vi "Load Subroutine Test Exec.vi"(4 "Path Builder":refnum<class "IPath Builder.lvclass">, 5 "Parallel in":refnum<class "Parallel.lvclass">, 6 "Persistence in":refnum<class "IPersist.lvclass">, 7 "Linked List ID":string, 8 "error in (no error)":errorcluster, 10 "Paths":path[](array[path]), 11 "Linked List Ref":refnum<data-value>) -> (0 "error out":errorcluster, 3 "Linked List Ref out":refnum<data-value>)   [LabVIEW 2017]
uses:
  Test Executive/ITestExecutive/ITest Executive.lvclass
  linked-list/Source/Linked List/Linked List Ref/Linked List Ref.lvclass
  b9c2613a-6aa9-4761-86d5-781f96568d67.vi
  Test Executive/TestExecutive Ref/TestExecutive Ref.lvclass
  cfb7364d-dae3-4f2b-ba87-61db7f054fd9.vi
  1f521296-bf4a-4187-b7fe-4ed0693accc0.vi
  8fd00299-f1f7-40b8-accc-d4ca8393805f.vi
  7c02b004-8b9d-45a5-be84-3e65cc974b1d.vi
  Test Executive Data Type/Test Executive.lvclass
  Custom Type Test Executive/Custom Type Test Executive.lvclass
  dc836278-d113-4003-92ad-fcb185286903.vi
  a563c450-6208-4c7f-b57f-94cea08b9ed5.vi
  6d463ee5-b5b8-463a-9b9c-645794412c76.vi
  data-type-serializer/source/Boolean/Boolean.lvclass
  data-type-serializer/source/String 1D/String 1D.lvclass
  Test Executive 1D Data Type/Test Executive 1D.lvclass
  C:/Users/jonmc/Documents/Git/Test Executive/gpm_packages/@cs/data-type-serializer/source/Data Type/Data Type.lvclass
  C:/Users/jonmc/Documents/Git/Test Executive/Source/Test Executive/ITestExecutive/ITest Executive.lvclass
  linked-list/Source/Linked List/ILinkedList/ILinked List.lvclass
  Path Builder/IPath Builder/IPath Builder.lvclass
  persistence/source/IPersist/IPersist.lvclass
  Parallel.lvclass
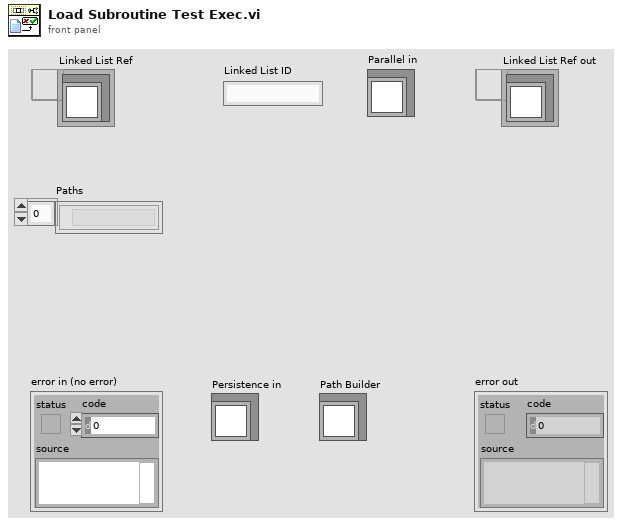
[diagram p1: front panel]
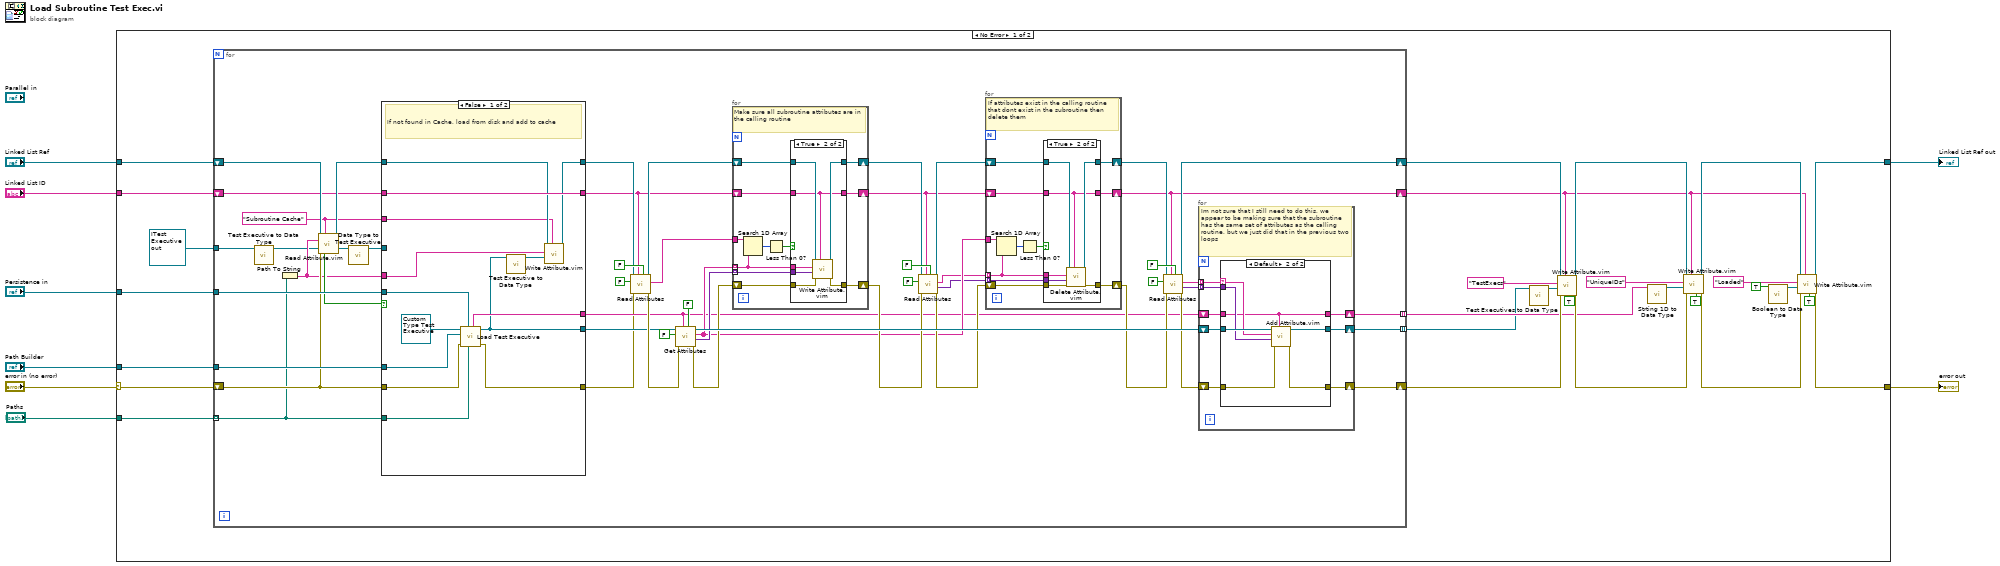
[diagram p0: block diagram]
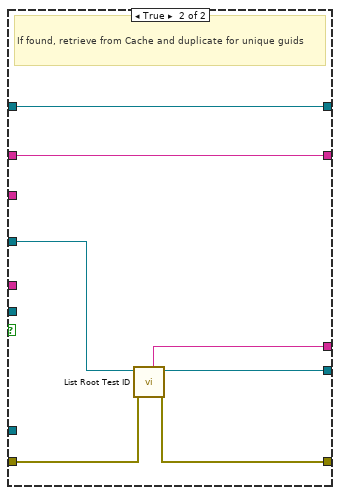
[diagram p2: hidden frame]
diagram:
  n1 = case shown="No Error" "error in (no error)" {
    selector: "error in (no error)" -> [w33 w169]
    tunnel: "Persistence in" -> [w36 _]
    tunnel: "Paths" -> [w32 _]
    tunnel: "Path Builder" -> [w35 _]
    tunnel: "Linked List Ref" -> [w34 w170]
    tunnel: "Linked List ID" -> [w31 _]
    tunnel: [w16 w170] -> w2
    tunnel: [w14 w169] -> w3
    frame No Error {
      n2 = for {
        tunnel: w36 -> [w87]
        tunnel: w35 -> [w86]
        tunnel: w32 -> [w54] mode=indexing
        tunnel: refnum<data-value> refnum ("Test Executive Ref out") -> [w48]
        shift-right: [w61] -> w17
        shift-left: w34 -> [w56]
        shift-right: [w84] -> w15
        shift-left: w33 -> [w55]
        shift-right: [w39] -> w13
        shift-left: w31 -> [w51]
        tunnel: [w38] -> w10 mode=indexing
        tunnel: [w37] -> w12 mode=indexing
        w49 = "Subroutine Cache" ("Name")
        n3 = call "Test Executive to Data Type.vi"("Test Executive Ref"=w48) -> ("Boolean out"=w47:refnum<class "Test Executive.lvclass">)  [unwired: 9 in, 1 out]
        n4 = Path To String(path=w54) -> (string=w50:string)
        n5 = call "Read Attribute.vim"("Linked List Ref"=w56, "Linked List ID"=w49, "Attribute Name"=w50, "Type"=w47, "error in (no error)"=w55) -> ("Linked List Ref out"=w52:refnum<data-value>, "Attribute"=w46:refnum<class "Test Executive.lvclass">, "Found?"=w53:bool)  [unwired: 5 in, 3 out]
        n6 = call "Data Type to Test Executive.vi"("Data Type"=w46) -> ("Test Executive Ref"=w45:refnum<data-value>)  [unwired: 9 in, 1 out]
        n7 = case shown="False" w53 {
          tunnel: [w101 w105] -> w40
          tunnel: w87 -> [w100 _]
          tunnel: w86 -> [w99 _]
          tunnel: [w90 w103] -> w41
          tunnel: [w91 w102] -> w42
          tunnel: w55 -> [w98 w106]
          tunnel: w54 -> [w97 _]
          tunnel: [w94 w108] -> w44
          tunnel: w52 -> [w95 w108]
          tunnel: [w96 w107] -> w43
          tunnel: w51 -> [w96 w107]
          tunnel: w50 -> [w92 _]
          tunnel: w49 -> [w93 _]
          tunnel: w45 -> [_ w104]
          frame False {
            # "If not found in Cache, load from disk and add to cache"
            n8 = call "Load Test Executive.vi"("Folder"=w97, "Persistence in"=w100, "error in (no error)"=w98, "Path Builder"=w99, "Test Executive"=refnum<class "Custom Type Test Executive.lvclass"> refnum ("Custom Type Test Executive.lvlib:Custom Type Test Executive.lvclass")) -> ("error out"=w101:errorcluster, "Test Executive Ref out"=w90:refnum<data-value>, "Root ID"=w91:string)  [unwired: 4 in]
            n9 = call "Test Executive to Data Type.vi"("Test Executive Ref"=w90) -> ("Boolean out"=w89:refnum<class "Test Executive.lvclass">)  [unwired: 9 in, 1 out]
            n10 = call "Write Attribute.vim"("Linked List ID"=w93, "Attribute"=w89, "Attribute Name"=w92, "Linked List Ref"=w95) -> ("Linked List Ref out"=w94:refnum<data-value>)  [unwired: 4 in, 3 out]
          }
          frame True {
            # "If found, retrieve from Cache and duplicate for unique guids"
            n11 = call "List Root Test ID.vi"("error in (no error)"=w106, "Test Executive Ref"=w104) -> ("error out"=w105:errorcluster, "Test Executive Ref out"=w103:refnum<data-value>, "Root ID"=w102:string)  [unwired: 5 in, 2 out]
          }
        }
        n12 = call "Read Attributes.vi"("Flatten Pointer?"=FALSE, "Linked List ID"=w43, "error in (no error)"=w40, "Include Private?"=FALSE, "Linked List Ref"=w44) -> ("error out"=w79:errorcluster, "Attribute Names out"=w78:string[], "Linked List Ref out"=w76:refnum<data-value>)  [unwired: 1 in, 3 out]
        n13 = call "Get Attributes.vi"("Flatten Pointer?"=FALSE, "Test ID"=w42, "error in (no error)"=w79, "Include Private?"=FALSE, "Test Executive Ref"=w41) -> ("error out"=w75:errorcluster, "Attributes"=w77:variant[], "Attribute Names out"=w67:string[], "Test Executive Ref out"=w82:refnum<data-value>)  [unwired: 1 in, 2 out]
        n14 = for {
          tunnel: w67 -> [w132] mode=indexing
          tunnel: w77 -> [w131] mode=indexing
          shift-right: [w137] -> w71
          shift-left: w76 -> [w138]
          tunnel: w78 -> [w139]
          shift-right: [w135] -> w72
          shift-left: w75 -> [w136]
          shift-right: [w130] -> w69
          shift-left: w43 -> [w134]
          # "Make sure all subroutine attributes are in the calling routine"
          n15 = Search 1D Array(1D array=w139, element=w132) -> (index of element=w140:i32)  [unwired: 1 in]
          n16 = Less Than 0?(x=w140) -> (x < 0?=w133:bool)
          n17 = case shown="True" w133 {
            tunnel: w138 -> [w143 w150]
            tunnel: [w143 w149] -> w137
            tunnel: w136 -> [w142 w148]
            tunnel: [w142 w147] -> w135
            tunnel: w134 -> [w141 w144]
            tunnel: w132 -> [_ w146]
            tunnel: w131 -> [_ w145]
            tunnel: [w141 w144] -> w130
            frame False {
            }
            frame True {
              n18 = call "Write Attribute.vim"("Linked List ID"=w144, "error in (no error)"=w148, "Attribute"=w145, "Attribute Name"=w146, "Linked List Ref"=w150) -> ("error out"=w147:errorcluster, "Linked List Ref out"=w149:refnum<data-value>)  [unwired: 3 in, 2 out]
            }
          }
        }
        n19 = call "Read Attributes.vi"("Flatten Pointer?"=FALSE, "Linked List ID"=w69, "error in (no error)"=w72, "Include Private?"=FALSE, "Linked List Ref"=w71) -> ("error out"=w68:errorcluster, "Attributes"=w65:variant[], "Attribute Names out"=w66:string[], "Linked List Ref out"=w70:refnum<data-value>)  [unwired: 1 in, 2 out]
        n20 = for {
          tunnel: w66 -> [w111] mode=indexing
          tunnel: w65 -> [w110] mode=indexing
          shift-right: [w116] -> w62
          shift-left: w70 -> [w117]
          tunnel: w67 -> [w118]
          shift-right: [w114] -> w60
          shift-left: w68 -> [w115]
          shift-right: [w109] -> w39
          shift-left: w69 -> [w113]
          # "If attributes exist in the calling routine that dont exist in the subroutine then delete them"
          n21 = Search 1D Array(1D array=w118, element=w111) -> (index of element=w119:i32)  [unwired: 1 in]
          n22 = Less Than 0?(x=w119) -> (x < 0?=w112:bool)
          n23 = case shown="True" w112 {
            tunnel: w117 -> [w122 w129]
            tunnel: [w122 w128] -> w116
            tunnel: w115 -> [w121 w126]
            tunnel: [w121 w125] -> w114
            tunnel: w113 -> [w120 w127]
            tunnel: w111 -> [_ w124]
            tunnel: w110 -> [_ w123]
            tunnel: [w120 w127] -> w109
            frame False {
            }
            frame True {
              n24 = call "Delete Attribute.vim"("Linked List ID"=w127, "error in (no error)"=w126, "Type"=w123, "Attribute Name"=w124, "Linked List Ref"=w129) -> ("error out"=w125:errorcluster, "Linked List Ref out"=w128:refnum<data-value>)  [unwired: 4 in, 1 out]
            }
          }
        }
        n25 = call "Read Attributes.vi"("Flatten Pointer?"=FALSE, "Linked List ID"=w39, "error in (no error)"=w60, "Include Private?"=FALSE, "Linked List Ref"=w62) -> ("error out"=w59:errorcluster, "Attributes"=w58:variant[], "Attribute Names out"=w57:string[], "Linked List Ref out"=w61:refnum<data-value>)  [unwired: 1 in, 2 out]
        n26 = for {
          shift-right: [w155] -> w84
          shift-left: w59 -> [w156]
          tunnel: w57 -> [w154] mode=indexing
          tunnel: w58 -> [w153] mode=indexing
          shift-right: [w152] -> w37
          shift-left: w42 -> [w157]
          shift-right: [w151] -> w38
          shift-left: w82 -> [w158]
          # "Im not sure that I still need to do this, we appear to be making sure that the subroutine has the same set of attributes as the calling routine, but we just did that in the previous two loops"
          n27 = case shown="Default" w154 {
            selector: w154 -> [_ w165]
            tunnel: w158 -> [w159 w168]
            tunnel: w157 -> [w160 w163]
            tunnel: w156 -> [w161 w167]
            tunnel: [w161 w166] -> w155
            tunnel: w153 -> [_ w164]
            tunnel: [w160 w163] -> w152
            tunnel: [w159 w162] -> w151
            frame "Restore Point" {
            }
            frame Default {
              n28 = call "Add Attribute.vim"("ID"=w163, "error in (no error)"=w167, "Attribute"=w164, "Attribute Name"=w165, "Test Executive Ref"=w168) -> ("error out"=w166:errorcluster, "Test Executive Ref out"=w162:refnum<data-value>)  [unwired: 3 in, 2 out]
            }
          }
        }
      }
      n29 = call "Test Executives to Data Type.vi"("Test Executive Refs"=w10) -> ("Boolean out"=w9:refnum<class "Test Executive 1D.lvclass">)  [unwired: 9 in, 1 out]
      n30 = call "Write Attribute.vim"("Private?"=TRUE, "Linked List ID"=w13, "error in (no error)"=w15, "Attribute"=w9, "Attribute Name"="TestExecs", "Linked List Ref"=w17) -> ("error out"=w26:errorcluster, "Linked List Ref out"=w21:refnum<data-value>)  [unwired: 2 in, 2 out]
      n31 = call "Strting 1D to Data Type.vi"("String 1D"=w12) -> ("Boolean out"=w11:refnum<class "String 1D.lvclass">)  [unwired: 9 in, 1 out]
      n32 = call "Write Attribute.vim"("Private?"=TRUE, "Linked List ID"=w13, "error in (no error)"=w26, "Attribute"=w11, "Attribute Name"="UniqueIDs", "Linked List Ref"=w21) -> ("error out"=w23:errorcluster, "Linked List Ref out"=w20:refnum<data-value>)  [unwired: 2 in, 2 out]
      n33 = call "Boolean to Data Type.vi"("Boolean"=TRUE) -> ("Boolean out"=w19:refnum<class "Boolean.lvclass">)  [unwired: 9 in, 1 out]
      n34 = call "Write Attribute.vim"("Private?"=TRUE, "Linked List ID"=w13, "error in (no error)"=w23, "Attribute"=w19, "Attribute Name"="Loaded", "Linked List Ref"=w20) -> ("error out"=w14:errorcluster, "Linked List Ref out"=w16:refnum<data-value>)  [unwired: 2 in, 2 out]
    }
    frame Error {
    }
  }
  "error out" <- w3
  "Linked List Ref out" <- w2
